vi "Evaluate Interpolating Polynomial.vi"(9 "xi":dbl[](array[numeric]) format="%_6g", 11 "piecewise polynomial":T1 {"x locations" format="%.4g"; "coefficients" format="%.4g"}) -> (0 "error":i32, 3 "yi":dbl[](array[numeric]) format="%_6g")   [LabVIEW 2014, in "NI_Gmath.lvlib"]
doc: "Takes the <B>piecewise polynomial</B> cluster and computes the interpolated values <B>yi</B> at each <B>xi</B> location."
uses:
  NI_Gmath.lvlib
  in_piecewise interp poly control.ctl
  Scalar Polynomial Evaluation (DBL).vi
  NI_AALPro.lvlib
panel:
  # "Evaluate Interpolating Polynomial"
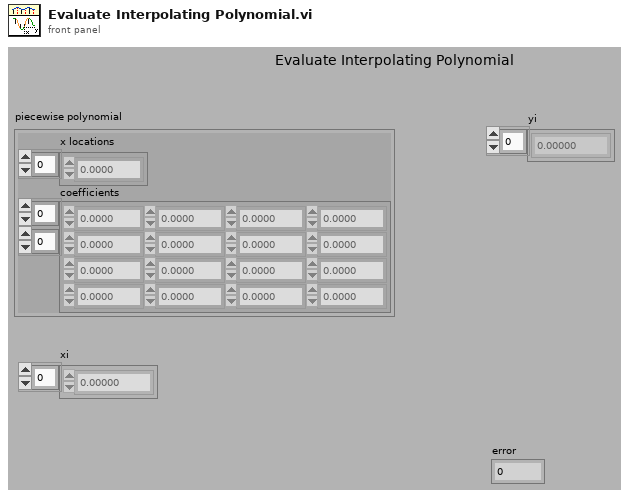
[diagram p1: front panel]
types:
  T1 = typedef "NI_Gmath.lvlib/in_piecewise interp poly control.ctl" = cluster{"x locations":dbl[], "coefficients":dbl[][]}
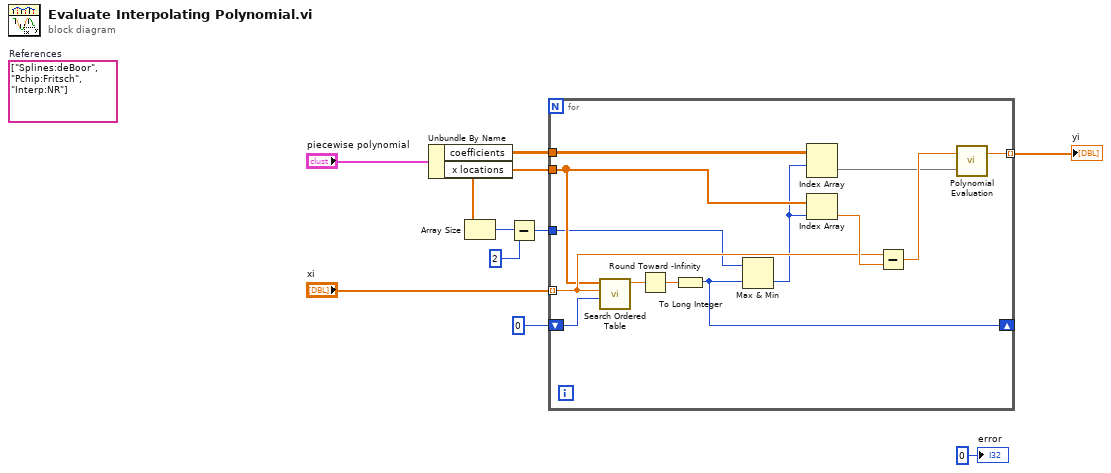
[diagram p0: block diagram]
diagram:
  (unwired) string[] ["Splines:deBoor", "Pchip:Fritsch", "Interp:NR"]  # References
  n1 = Unbundle By Name("piecewise polynomial") -> ("coefficients"=w9:dbl[][], "x locations"=w8:dbl[])
  n2 = Array Size(array=w8) -> (size(s)=w7:i32)
  n3 = Subtract(x=w7, y=2) -> (x-y=w5:i32)
  n4 = for {
    tunnel: w9 -> [w22]
    tunnel: "xi" -> [w17] mode=indexing
    tunnel: w8 -> [w15]
    tunnel: [w20] -> w3 mode=indexing
    tunnel: w5 -> [w12]
    shift-right: [w13] -> _
    shift-left: 0 -> [w16]
    n5 = call "Search Ordered Table.vi"("starting index"=w16, "x value"=w17, "ordered x array"=w15) -> ("fractional index"=w14:dbl)  [unwired: 8 in]
    n6 = Round Toward -Infinity(1:w14) -> (0:w18:dbl)
    n7 = To Long Integer(number=w18) -> (32bit integer=w13:i32)
    n8 = Max & Min(x=w12, y=w13) -> (min(x,y)=w11:i32)  [unwired: 1 out]
    n9 = Index Array(array=w22, index (row)=w11) -> (element=w19:dbl[])  [unwired: 1 in]
    n10 = Index Array(array=w15, index=w11) -> (element=w23:dbl)
    n11 = Subtract(x=w17, y=w23) -> (x-y=w21:dbl)
    n12 = call-poly "Polynomial Evaluation.vi"("P(x)"=w19, "a"=w21) -> ("P(a)"=w20:dbl)  [unwired: 1 out]
  }
  "yi" <- w3
  "error" <- 0 ("error")
